vi "Range Create.vi"(8 "error in (no error)":errorcluster, 9 "Delta value":refnum<data-value>, 10 "Ending":refnum<data-value>, 11 "Begin":refnum<data-value>) -> (0 "error out":errorcluster, 3 "Range DVR out":refnum<data-value>)   [LabVIEW 2010, in "MDSplus.lvlib"]
uses:
  <vilib>/MDSplus/Library/MDSplus.lvlib
  <vilib>/MDSplus/Classes/Data_Class/Compound_Class/Range_Class/Range.lvclass
  <vilib>/MDSplus/Classes/Data_Class/Data.lvclass
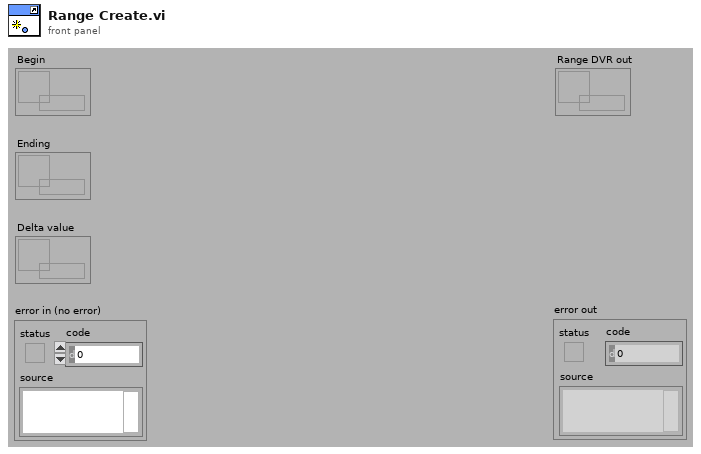
[diagram p1: front panel]
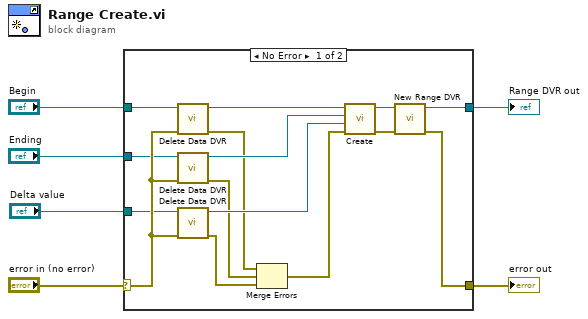
[diagram p0: block diagram]
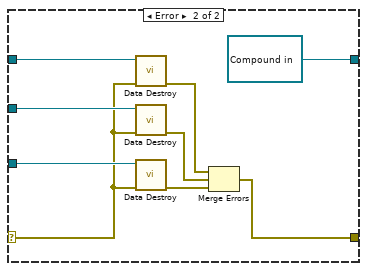
[diagram p2: hidden frame]
diagram:
  n1 = case shown="No Error" "error in (no error)" {
    selector: "error in (no error)" -> [w20 w27]
    tunnel: [w7 w23] -> w6
    tunnel: [w15 refnum<data-value> refnum ("Range DVR out")] -> w4
    tunnel: "Begin" -> [w21 w30]
    tunnel: "Ending" -> [w19 w29]
    tunnel: "Delta value" -> [w18 w28]
    frame No Error {
      n2 = call <vilib>:"Delete Data DVR.vi"("error in (no error)"=w20, "Data DVR in"=w21) -> ("error out"=w9:errorcluster, "Data out"=w14:refnum<class "Data.lvclass">)  [unwired: 8 in]
      n3 = call <vilib>:"Delete Data DVR.vi"("error in (no error)"=w20, "Data DVR in"=w19) -> ("error out"=w10:errorcluster, "Data out"=w13:refnum<class "Data.lvclass">)  [unwired: 8 in]
      n4 = call <vilib>:"Delete Data DVR.vi"("error in (no error)"=w20, "Data DVR in"=w18) -> ("error out"=w11:errorcluster, "Data out"=w12:refnum<class "Data.lvclass">)  [unwired: 8 in]
      n5 = Merge Errors(w9, w10, w11) -> (w8:errorcluster)
      n6 = call <vilib>:"Create.vi"("error in (no error)"=w8, "Delta value"=w12, "Ending"=w13, "Begin"=w14) -> ("error out"=w17:errorcluster, "Range out"=w16:refnum<class "Range.lvclass">)  [unwired: 6 in]
      n7 = call <vilib>:"New Range DVR.vi"("error in (no error)"=w17, "Range in"=w16) -> ("error out"=w7:errorcluster, "Range DVR out"=w15:refnum<data-value>)  [unwired: 8 in]
    }
    frame Error {
      n8 = call <vilib>:"Data Destroy.vi"("error in (no error)"=w27, "Data DVR in"=w30) -> ("error out"=w26:errorcluster)  [unwired: 9 in]
      n9 = call <vilib>:"Data Destroy.vi"("error in (no error)"=w27, "Data DVR in"=w29) -> ("error out"=w25:errorcluster)  [unwired: 9 in]
      n10 = call <vilib>:"Data Destroy.vi"("error in (no error)"=w27, "Data DVR in"=w28) -> ("error out"=w24:errorcluster)  [unwired: 9 in]
      n11 = Merge Errors(w26, w25, w24) -> (w23:errorcluster)
    }
  }
  "error out" <- w6
  "Range DVR out" <- w4
